vi "Is Command Complete.vi"(8 "error in (no error)":errorcluster, 11 "Command in":refnum<class "Command.lvclass">) -> (0 "error out":errorcluster, 3 "Command out":refnum<class "Command.lvclass">)   [LabVIEW 2013, in "Command.lvclass"]
uses:
  Command.lvclass
  Command.lvclass/Command.ctl
  States/State/State.lvclass
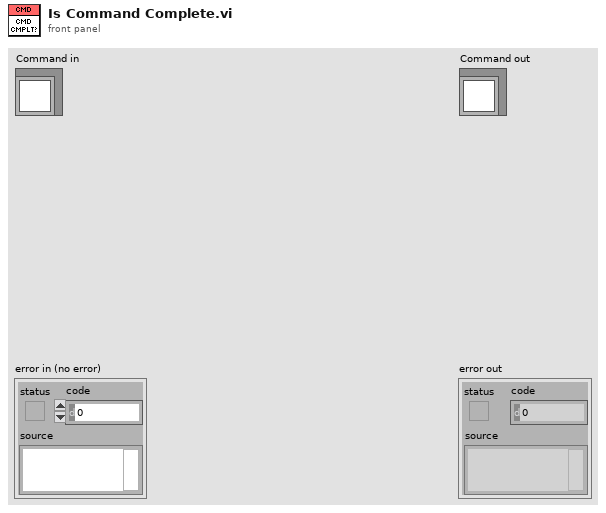
[diagram p1: front panel]
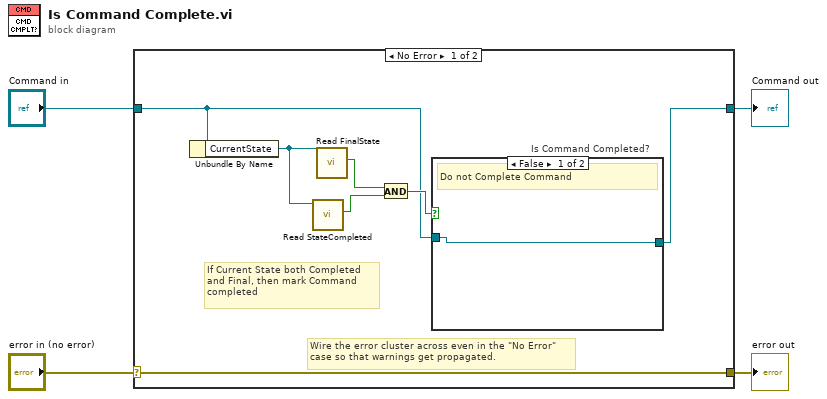
[diagram p0: block diagram]
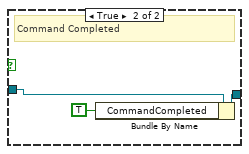
[diagram p2: hidden frame]
diagram:
  n1 = case shown="No Error" "error in (no error)" {
    selector: "error in (no error)" -> [w11 w17]
    tunnel: [w11 w17] -> w3
    tunnel: [w5 w16] -> w1
    tunnel: "Command in" -> [w6 w16]
    frame No Error {
      # "If Current State both Completed\nand Final, then mark Command \ncompleted"
      # "Wire the error cluster across even in the \"No Error\"\ncase so that warnings get propagated."
      n2 = Unbundle By Name(w6) -> ("CurrentState"=w10:refnum<class "State.lvclass">)
      n3 = call-dynamic "Read StateCompleted.vi"("State in"=w10) -> ("StateCompleted"=w8:bool)  [unwired: 8 in, 2 out]
      n4 = call-dynamic "Read FinalState.vi"("State in"=w10) -> ("FinalState"=w9:bool)  [unwired: 8 in, 2 out]
      n5 = And(x=w9, y=w8) -> (x .and. y?=w7:bool)
      n6 = case "Is Command Completed?" shown="False" w7 {
        tunnel: w6 -> [w12 w15]
        tunnel: [w12 w14] -> w5
        frame False {
          # "Do not Complete Command"
        }
        frame True {
          # "Command Completed"
          n7 = Bundle By Name(cluster=w15, "CommandCompleted"=TRUE) -> (w14:refnum<class "Command.lvclass">)
        }
      }
    }
    frame Error {
    }
  }
  "error out" <- w3
  "Command out" <- w1
